vi "Get_Vector_Angle.vi"(10 "End Point":cluster{"X":dbl, "Y":dbl}, 11 "Start Point":cluster{"X":dbl, "Y":dbl}) -> (3 "Angle Out":dbl)   [LabVIEW 2014]
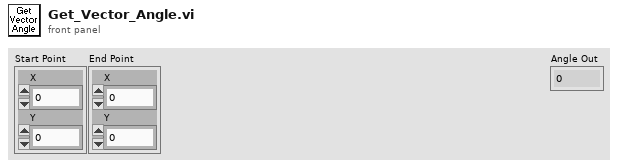
[diagram p1: front panel]
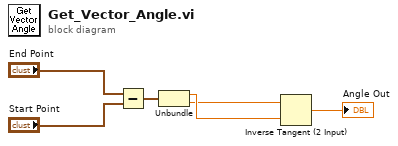
[diagram p0: block diagram]
diagram:
  n1 = Subtract(x="End Point", y="Start Point") -> (x-y=w4:cluster{"X":dbl, "Y":dbl})
  n2 = Unbundle(w4) -> ("X"=w3:dbl, "Y"=w2:dbl)
  n3 = Inverse Tangent (2 Input)(1:w3, 2:w2) -> (0:→"Angle Out":dbl)
